vi "EditValue.vi"(8 "error in (no error)":errorcluster, 10 "Bounds":T1, 11 "COM Port D Element in":refnum<class "COM Port D Element.lvclass">) -> (0 "error out":errorcluster, 1 "Tabbed out?":bool, 2 "Value changed?":bool, 3 "COM Port D Element out":refnum<class "COM Port D Element.lvclass">)   [LabVIEW 2018, in "D Datagrid Library.lvlib" / "COM Port D Element.lvclass"]
uses:
  COM Port D Element.lvclass
  C:/dev/D Datagrid/String Dropdown D Element/String dropdown D Element.lvclass
  <vilib>/Utility/miscctls.llb/LVRectTypeDef.ctl
  <vilib>/Instr/_visa.llb/VISA Find Search Mode.ctl
  String Dropdown D Element/String dropdown D Element.lvclass/String dropdown D Element.ctl
  String Dropdown D Element/Write Strings.vi
  String Dropdown D Element/String dropdown D Element.lvclass
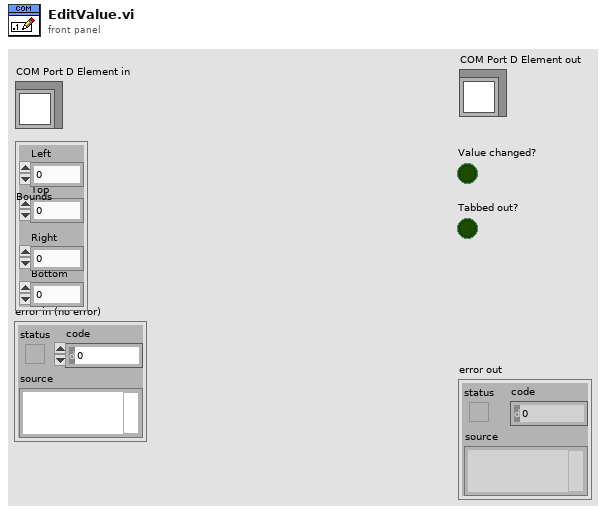
[diagram p1: front panel]
types:
  T1 = typedef "LVRectTypeDef.ctl" = cluster{"Left":i16, "Top":i16, "Right":i16, "Bottom":i16}
  T2 = typedef "VISA Find Search Mode.ctl" = u32
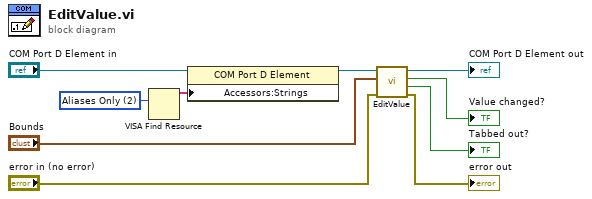
[diagram p0: block diagram]
diagram:
  w3 = T2 2 items=["Canonical Names Only"=0, "Aliases Only"=2, "Include Matching Aliases"=3, "Include All Aliases"=4] ("Search Mode")
  n1 = VISA Find Resource(10:w3) -> (3:w2:string[])  [unwired: 2 in, 2 out]
  n2 = property class="COM Port D Element"(reference="COM Port D Element in", "Accessors:Strings"=w2) -> (reference out=w8:refnum<class "COM Port D Element.lvclass">)  [unwired: 1 in, 1 out]
  n3 = call-parent "EditValue.vi"("error in (no error)"="error in (no error)", "Bounds"="Bounds", "Dropdown D Element in"=w8) -> ("error out"=→"error out":errorcluster, "Tabbed out?"=→"Tabbed out?":bool, "Value changed?"=→"Value changed?":bool, "Dropdown D Element out"=→"COM Port D Element out":refnum<class "COM Port D Element.lvclass">)  [unwired: 5 in]
